vi "Start Disconnect.vi"(8 "error in (no error)":errorcluster, 11 "TCP Comm":T1) -> (0 "error out":errorcluster)   [LabVIEW 2020, in "TinyTCP.lvlib"]
uses:
  TinyTCP.lvlib
  Instance.ctl
  Ref Data.ctl
  State.ctl
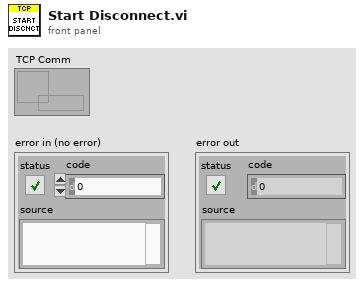
[diagram p1: front panel]
types:
  T1 = typedef "TinyTCP.lvlib/Instance.ctl" = refnum<data-value>
  T2 = typedef "TinyTCP.lvlib/State.ctl" = enum16{"Idle", "Starting", "Connecting", "Connected", "Disconnecting", "Stopped"}
  T3 = typedef "TinyTCP.lvlib/Ref Data.ctl" = cluster{"TCP":refnum<k5>, "State":T2, "Server":bool, "Host":string, "Port":u16, "Listener":refnum<k5>, "Start":bool, "Disconnect":bool, "TCP Valid":bool, "TLS Enabled":bool, "Immutable TLS":refnum<k36>, "Certificate DN":string, "local-port":u16}
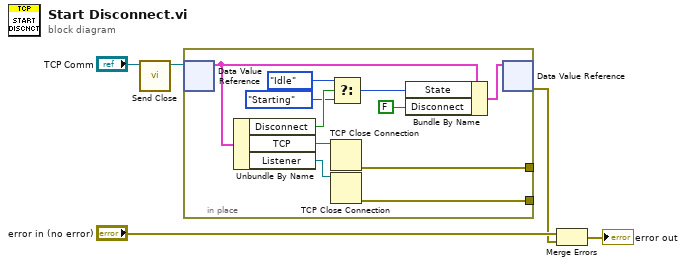
[diagram p0: block diagram]
diagram:
  n1 = call "Send Close.vi"("TCP Comm In"="TCP Comm") -> ("TCP Comm"=w1:T1)  [unwired: 9 in, 1 out]
  n2 = in-place {
    in-place-border: [w7] -> _
    in-place-border: [w6] -> _
    n3 = in-place-dvr #1(w1) -> (w14:T3)  [unwired: 1 out]
    n4 = Unbundle By Name(w14) -> ("Disconnect"=w10:bool, "TCP"=w12:refnum<k5>, "Listener"=w13:refnum<k5>)
    n5 = TCP Close Connection(connection ID=w12) -> (error out=w7:errorcluster)  [unwired: 2 in, 1 out]
    n6 = TCP Close Connection(connection ID=w13) -> (error out=w6:errorcluster)  [unwired: 2 in, 1 out]
    n7 = Select(t=State."Idle" ("State"), s=w10, f=State."Starting") -> (s? t:f=w8:T2)
    n8 = Bundle By Name(cluster=w14, "State"=w8, "Disconnect"=FALSE) -> (w16:T3)
    n9 = in-place-dvr #1(w16) -> (w4:errorcluster)  [unwired: 1 out]
  }
  n10 = Merge Errors("error in (no error)", w4) -> (→"error out":errorcluster)
